vi "update position and status to DB.vi"(7 "positions":dbl[](array[numeric]), 8 "error in (no error)":errorcluster, 9 "Array in":i32[](array[numeric]), 10 "VISA resource name in":refnum<visa-resource-name>, 11 "ESP301 in":refnum<class "ESP301.lvclass">) -> (0 "error out":errorcluster, 1 "motor Status":T1(array[ring]), 2 "VISA resource name out out":refnum<visa-resource-name>, 3 "ESP301 out":refnum<class "ESP301.lvclass">)   [LabVIEW 2020, in "ESP301.lvclass"]
uses:
  ESP301.lvclass
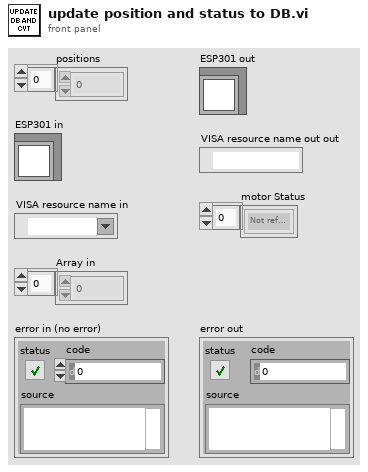
[diagram p1: front panel]
types:
  T1 = enum16{"Not referenced", "Homing", "Moving", "Ready"}[]
  T2 = enum16{"Not referenced", "Homing", "Moving", "Ready"}
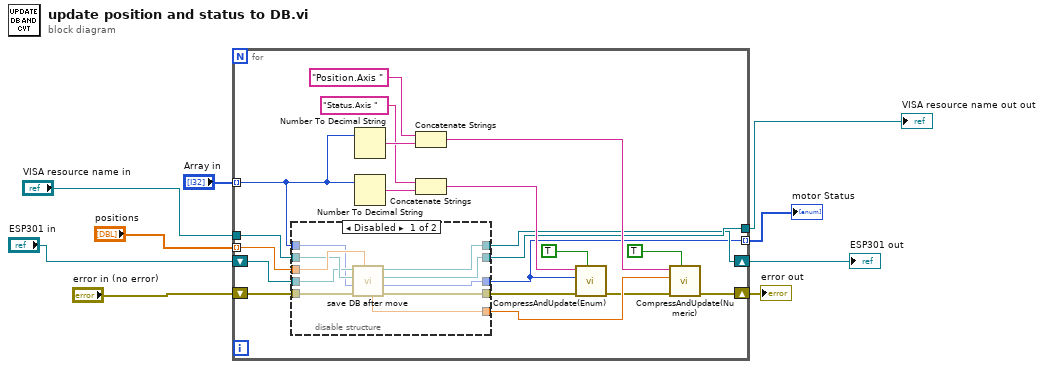
[diagram p0: block diagram]
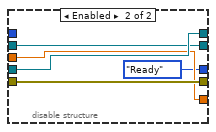
[diagram p2: hidden frame]
diagram:
  n1 = for {
    tunnel: [w19] -> w2
    tunnel: "Array in" -> [w14] mode=indexing
    tunnel: "positions" -> [w18] mode=indexing
    shift-right: [w16] -> w6
    shift-left: "ESP301 in" -> [w17]
    tunnel: "VISA resource name in" -> [w15]
    tunnel: [w12] -> w9 mode=indexing
    shift-right: [w10] -> w1
    shift-left: "error in (no error)" -> [w13]
    n2 = disable-structure shown="Disabled" {
      disable-tunnel: w13 -> [w39 w42]
      disable-tunnel: [w38 w41] -> w21
      disable-tunnel: [w37 T2."Ready" ("Axis 3")] -> w12
      disable-tunnel: w18 -> [w36 w41]
      disable-tunnel: [w35 w44] -> w16
      disable-tunnel: [w34 w42] -> w20
      disable-tunnel: w15 -> [w33 w43]
      disable-tunnel: w17 -> [w32 w44]
      disable-tunnel: [w31 w43] -> w19
      disable-tunnel: w14 -> [w30 _]
      frame Disabled {
        n3 = call-dynamic "save DB after move.vi"("Position (units) in"=w36, "error in (no error)"=w39, "Axis"=w30, "VISA resource name out in"=w33, "ESP301 in"=w32) -> ("error out"=w34:errorcluster, "Axis Status"=w37:T2, "VISA resource name out out"=w31:refnum<visa-resource-name>, "ESP301 out"=w35:refnum<class "ESP301.lvclass">, "Position (units) out"=w38:dbl)  [unwired: 2 in]
      }
      frame Enabled {
      }
    }
    n4 = Number To Decimal String(number=w14) -> (decimal integer string=w26:string)  [unwired: 1 in]
    n5 = Number To Decimal String(number=w14) -> (decimal integer string=w23:string)  [unwired: 1 in]
    n6 = Concatenate Strings("Position.Axis " ("command or variable name"), w26) -> (w25:string)
    n7 = Concatenate Strings("Status.Axis " ("command or variable name"), w23) -> (w22:string)
    n8 = call "CompressAndUpdate(Enum).vi"("force CVT update (false)"=TRUE, "error in"=w20, "enum variant"=w12, "command or variable name"=w22) -> ("error out"=w11:errorcluster)  [unwired: 7 in]
    n9 = call "CompressAndUpdate(Numeric).vi"("force CVT update (false)"=TRUE, "error in"=w11, "Numeric"=w21, "command or variable name"=w25) -> ("error out"=w10:errorcluster)  [unwired: 7 in]
  }
  "motor Status" <- w9
  "ESP301 out" <- w6
  "VISA resource name out out" <- w2
  "error out" <- w1
